vi "LRC-8.vi"(11 "string":string) -> (2 "LRC-8":u8, 3 "string with LRC-8":string)   [LabVIEW 2015, in "PL Modbus Client.lvclass"]
doc: "Calculates LRC-8 and appends it to <B>string</B>."
uses:
  PL Modbus Client.lvclass
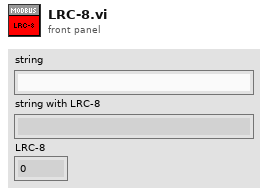
[diagram p1: front panel]
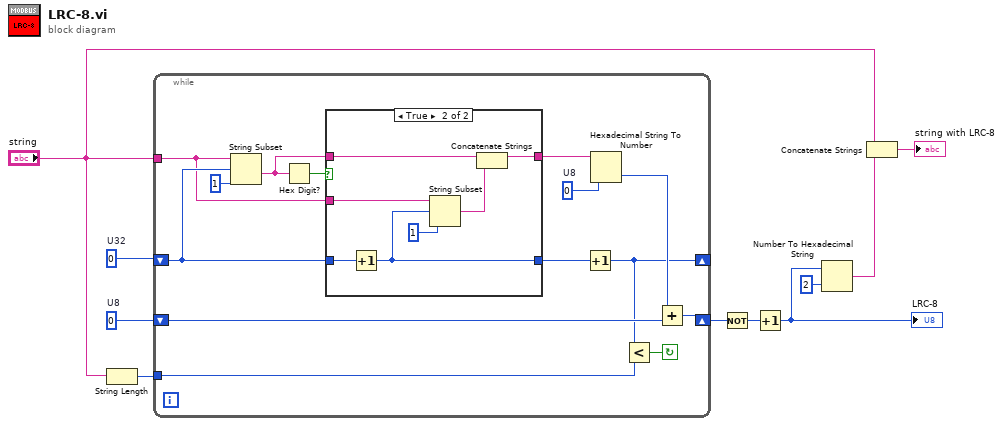
[diagram p0: block diagram]
diagram:
  w10 = u32 0  # U32
  w9 = u8 0  # U8
  n1 = String Length(string="string") -> (length=w8:i32)
  n2 = while {
    tunnel: "string" -> [w19]
    tunnel: w8 -> [w12]
    shift-left: w9 -> [w16]
    shift-right: [w15] -> w7
    shift-left: w10 -> [w23]
    shift-right: [w11] -> _
    stop <- w13 continue-if-true
    w18 = u8 0  # U8
    n3 = String Subset(string=w19, offset (0)=w23, length (rest)=1) -> (substring=w20:string)
    n4 = Hex Digit?(1:w20) -> (0:w21:bool)
    n5 = case shown="True" w21 {
      tunnel: w23 -> [w25 w33]
      tunnel: [w25 w31] -> w22
      tunnel: w20 -> [w26 w29]
      tunnel: w19 -> [_ w30]
      tunnel: [w26 w27] -> w17
      frame False {
      }
      frame True {
        n6 = Increment(x=w33) -> (x+1=w31:u32)
        n7 = String Subset(string=w30, offset (0)=w31, length (rest)=1) -> (substring=w28:string)
        n8 = Concatenate Strings(w29, w28) -> (w27:string)
      }
    }
    n9 = Increment(x=w22) -> (x+1=w11:u32)
    n10 = Hexadecimal String To Number(string=w17, default (0uL)=w18) -> (number=w14:u8)  [unwired: 2 out]
    n11 = Less?(x=w11, y=w12) -> (x < y?=w13:bool)
    n12 = Add(x=w14, y=w16) -> (x+y=w15:u8)
  }
  n13 = Not(x=w7) -> (.not. x?=w6:u8)
  n14 = Increment(x=w6) -> (x+1=w1:u8)
  "LRC-8" <- w1
  n15 = Number To Hexadecimal String(1:i16 2 ("width (-)"), 2:w1) -> (0:w5:string)
  n16 = Concatenate Strings("string", w5) -> (→"string with LRC-8":string)
